vi "fpga_Calculate Timestamp (P Class).vi"(0 "resample data and position":T2 {"frequency" format="%.59g"; "Resample position" format="%.53g"; "even-angle signal" format="%.30g"}, 1 "timestamp&count":T4 {"TAI timestamp" format="%.42g"}, 7 "muti_ch position valid?":bool, 9 "input valid":bool, 11 "Fnom":T1 items=["Fnom=50Hz", "Fnom=60Hz"], 12 "ready for output":bool) -> (4 "Resample data and time":T3, 6 "freq time difference":fxp<+,18,-4>, 10 "output valid":bool, 14 "ready for input":bool)   [LabVIEW 2013, in "NI_EP_PMU_FPGA.lvlib"]
uses:
  <vilib>/addons/Electrical Power/PMU/NI_EP_PMU_FPGA.lvlib
  <vilib>/addons/Electrical Power/PQ/Resampling/FPGA/subVIs/fpga_Resampled.ctl
  <vilib>/addons/Electrical Power/PQ/Resampling/FPGA/subVIs/fpga_Typedef Fnom.ctl
  <vilib>/rvi/FXPMathLib/basic elements/FxpDiscreteDelay/XNode/nifxpmath_DiscreteDelay.xnode
  <vilib>/rvi/FXPMathLib/FxpSub/XNode/nifxpmath_Sub.xnode
  <vilib>/rvi/FXPMathLib/FxpMul/XNode/nifxpmath_Multiplier.xnode
  <vilib>/addons/Electrical Power/PQ/Resampling/NI_EP_Resample_FPGA.lvlib
  <vilib>/rvi/FXPMathLib/sim/FxpSim.dll
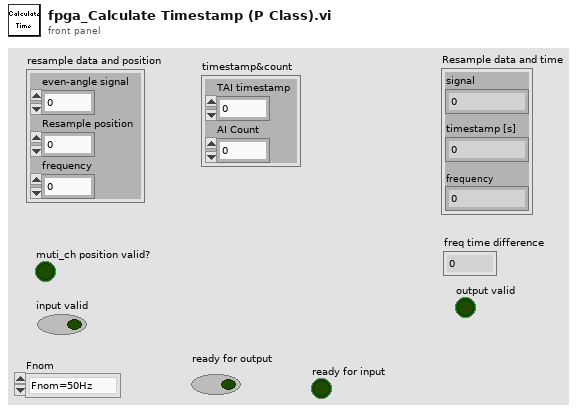
[diagram p1: front panel]
types:
  T1 = typedef "NI_EP_Resample_FPGA.lvlib/fpga_Typedef Fnom.ctl" = u8
  T2 = cluster{"even-angle signal":fxp<+/-,32,3>, "Resample position":fxp<+,64,16>, "frequency":fxp<+,32,8>}
  T3 = typedef "NI_EP_Resample_FPGA.lvlib/fpga_Resampled.ctl" = cluster{"signal":fxp<+/-,32,3>, "timestamp [s]":fxp<+,64,32>, "frequency":fxp<+,32,8>}
  T4 = cluster{"TAI timestamp":fxp<+,64,32>, "AI Count":u16}
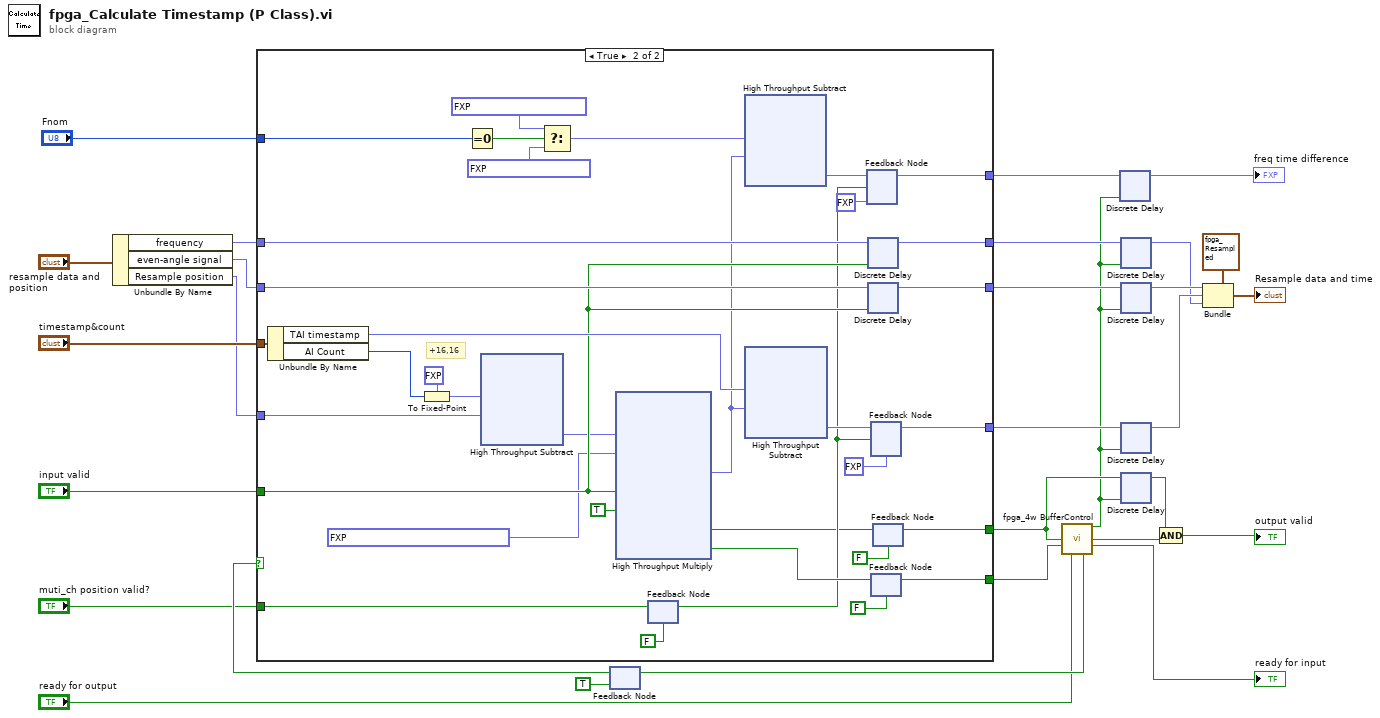
[diagram p0: block diagram]
diagram:
  n1 = Unbundle By Name("resample data and position") -> ("frequency"=w8:fxp<+,32,8>, "even-angle signal"=w7:fxp<+/-,32,3>, "Resample position"=w6:fxp<+,64,16>)
  n2 = feedback #1(TRUE ("logic enable")) -> (w27:bool)
  n3 = case shown="True" w27 {
    tunnel: "timestamp&count" -> [_ w55]
    tunnel: w7 -> [_ w45]
    tunnel: w6 -> [_ w54]
    tunnel: w8 -> [_ w47]
    tunnel: "input valid" -> [_ w43]
    tunnel: "muti_ch position valid?" -> [_ w53]
    tunnel: [_ w52] -> w14
    tunnel: [_ w49] -> w18
    tunnel: [_ w46] -> w17
    tunnel: [_ w44] -> w16
    tunnel: [_ w48] -> w15
    tunnel: "Fnom" -> [_ w37]
    tunnel: [_ w33] -> w2
    frame False {
    }
    frame True {
      # "+16,16"
      n4 = Unbundle By Name(w55) -> ("TAI timestamp"=w62:fxp<+,64,32>, "AI Count"=w56:u16)
      n5 = To Fixed-Point(fixed-point type=fxp<+,16,16> 0.0, number=w56) -> (fixed-point=w63:fxp<+,16,16>)
      n6 = Equal To 0?(x=w37) -> (x = 0?=w38:bool)
      n7 = xnode "High Throughput Subtract"("x"=w63, "y"=w54) -> ("x-y"=w41:fxp<+,32,16>)
      n8 = Select(t=fxp<+,18,-4> 0.010560035705566406 ("y"), s=w38, f=fxp<+,18,-4> 0.009059906005859375 ("y")) -> (s? t:f=w36:fxp<+,18,-4>)
      n9 = xnode ("High Throughput Multiply")("x"=w41, "y"=fxp<+,16,-15> 2.00001522898674e-05 ("Numeric"), "input valid"=w43, "ready for output (T)"=TRUE) -> ("x*y"=w30:fxp<+,64,32>, "output valid"=w31:bool, "ready for input"=w50:bool)
      n10 = feedback #2(FALSE ("muti_ch position valid?")) -> (w32:bool)
      n11 = feedback-in #2(w53) -> ()
      n12 = xnode "High Throughput Subtract"("x"=w36, "y"=w30) -> ("x-y"=w35:fxp<+,18,-4>)
      n13 = xnode "High Throughput Subtract"("x"=w62, "y"=w30) -> ("x-y"=w60:fxp<+,64,32>)
      n14 = feedback #3(fxp<+,18,-4> 0.0 ("y")) -> (w33:fxp<+,18,-4>)
      n15 = feedback-in #3(w35, w32) -> ()
      n16 = xnode ("Discrete Delay")("D"=w47, "enable"=w43) -> ("Q"=w46:fxp<+,32,8>)
      n17 = xnode ("Discrete Delay")("D"=w45, "enable"=w43) -> ("Q"=w44:fxp<+/-,32,3>)
      n18 = feedback #4(fxp<+,64,32> 0.0 ("x-y")) -> (w48:fxp<+,64,32>)
      n19 = feedback-in #4(w60, w32) -> ()
      n20 = feedback #5(FALSE ("output valid")) -> (w49:bool)
      n21 = feedback-in #5(w50) -> ()
      n22 = feedback #6(FALSE ("output valid")) -> (w52:bool)
      n23 = feedback-in #6(w31) -> ()
    }
  }
  n24 = call <vilib>:"fpga_4w BufferControl.vi"("DR"=w14, "RFI"=w18, "RFO"="ready for output") -> ("buff enable"=w3:bool, "output valid"=w24:bool, "ready for input"=→"ready for input":bool, "logic enable"=w29:bool)  [unwired: 9 in]
  n25 = feedback-in #1(w29) -> ()
  n26 = xnode ("Discrete Delay")("D"=w2, "enable"=w3) -> ("Q"=→"freq time difference":fxp<+,18,-4>)
  n27 = xnode ("Discrete Delay")("D"=w17, "enable"=w3) -> ("Q"=w11:fxp<+,32,8>)
  n28 = xnode ("Discrete Delay")("D"=w16, "enable"=w3) -> ("Q"=w13:fxp<+/-,32,3>)
  n29 = xnode ("Discrete Delay")("D"=w15, "enable"=w3) -> ("Q"=w12:fxp<+,64,32>)
  n30 = xnode ("Discrete Delay")("D"=w14, "enable"=w3) -> ("Q"=w26:bool)
  n31 = Compound Arithmetic op=AND(w26, w24) -> (→"output valid":bool)
  n32 = Bundle(cluster=T3 {"signal"=0.0, "timestamp [s]"=0.0, "frequency"=0.0} ("Resample data and time"), "signal"=w13, "timestamp [s]"=w12, "frequency"=w11) -> (→"Resample data and time":T3)
